vi "PrintScreen.vi"() -> ()   [LabVIEW 2016]
doc: "This code was originally designed to implement a PRINT SCREEN function. If run in its default state, the code simulates a PrintScreen keystroke. When executed, it gives you the option to take a screen capture of the active window (Alt-PrintScreen) or of the entire screen (PrintScreen). I added functionality to choose the keystroke you wish to simulate. It must be noted that the API call for some of the function may or may not cause minor inconvenient responses in the Window's environment. The added options were added solely to show the user how to make various API calls."
uses:
  <vilib>/picture/picture.llb/imagedata.ctl
  user32.dll
panel:
  out "y":u32
  out "x-y":u32
  out "Image":T1(plugin-control)
  in  "Keyboard Stroke 2":T2(ring)=enum."PRINT SCREEN"
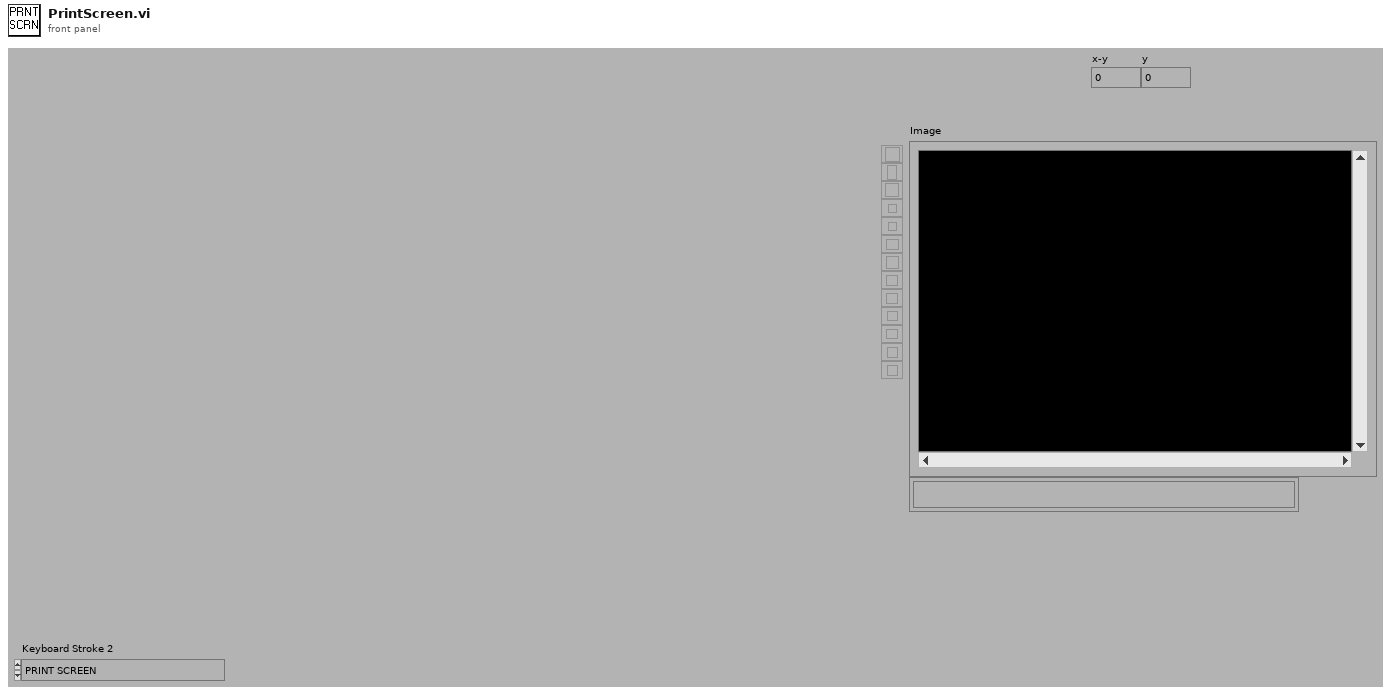
[diagram p1: front panel]
types:
  T1 = typedef "IMAQ Image.ctl" = refnum<image>
  T2 = enum16{"Left Mouse Button", "Right Mouse Button", "Ctrl-Break", "Middle Mouse Button (3-button mice only)", "X1 mouse button (Win2k Only)", "X2 Mouse Button (Win2k Only)", "Undefined (1)", "BACKSPACE", "TAB", "Reserved (1)", "Reserved (2)", "CLEAR", "ENTER", "Undefined (2)", "Undefined (3)", "SHIFT", "CTRL", "ALT", "PAUSE", "CAPS LOCK", "IME Kana mode", "Undefined (4)", "IME Junja mode", "IME final mode", "IME Hanja mode", "IME Kanji mode", "Undefined    ", "ESC", "IME convert", "IME nonconvert", "IME accept", "IME mode change request", "SPACEBAR", "PAGE UP", "PAGE DOWN", "END", "HOME", "LEFT ARROW", "UP ARROW", "RIGHT ARROW", "DOWN ARROW", "SELECT", "PRINT", "EXECUTE", "PRINT SCREEN", "INS", "DEL", "HELP"}
  T3 = typedef "imagedata.ctl" = cluster{"image type":i32, "image depth":i32, "image":u8[], "mask":u8[], "colors":u32[], "Rectangle":cluster{"left":i16, "top":i16, "right":i16, "bottom":i16}}
  T4 = typedef "Image Type" = u32
  T5 = typedef "LVRectTypeDef.ctl" = cluster{"left":i16, "top":i16, "right":i16, "bottom":i16}
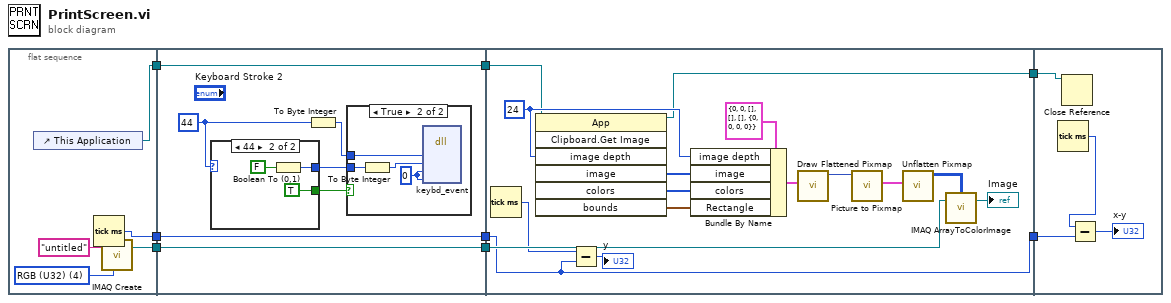
[diagram p0: block diagram]
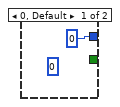
[diagram p3: hidden frame]
diagram:
  n1 = flat-sequence {
    tunnel: [w13] -> w7
    tunnel: [w10] -> w4
    tunnel: [w9] -> w2
    tunnel: [w16] -> w8
    tunnel: w7 -> [w16]
    tunnel: [w15] -> w5
    tunnel: w4 -> [w15]
    tunnel: [w14] -> w3
    tunnel: w2 -> [w14]
    tunnel: w8 -> [w30]
    tunnel: [w30] -> w6
    tunnel: w5 -> [w34]
    tunnel: w3 -> [w33]
    tunnel: [w32] -> w1
    tunnel: w6 -> [w48]
    tunnel: w1 -> [w45]
    frame #0 {
      w12 = T4 4 items=["Grayscale (U8)", "Grayscale (I16)", "Grayscale (SGL)", "Complex (CSG)", "RGB (U32)", "HSL (U32)", "RGB (U64)", "Grayscale (U16)"] ("Image Type")
      n2 = control-ref of="This Application"() -> (w9:refnum<vi>)
      n3 = Tick Count (ms)() -> (millisecond timer value=w13:u32)
      n4 = call "IMAQ Create"("Image Name"="untitled", "Image Type"=w12) -> ("New Image"=w10:T1)  [unwired: 3 in, 1 out]
    }
    frame #1 {
      w17 = 44
      n5 = case shown="44" w17 {
        tunnel: [i16 0 w28] -> w19
        tunnel: [_ TRUE ("T button?")] -> w18
        frame 0, Default {
          (unwired) i16 0
        }
        frame 44 {
          n6 = Boolean To (0,1)(Boolean=FALSE ("T button?")) -> (0, 1=w28:i16)
        }
      }
      n7 = To Byte Integer(number=w17) -> (8bit integer=w20:i8)
      n8 = case shown="True" w18 {
        tunnel: w19 -> [_ w22]
        tunnel: w20 -> [_ w21]
        frame False {
        }
        frame True {
          w23 = 0 ("Input Value")
          n9 = To Byte Integer(number=w22) -> (8bit integer=w24:i8)
          n10 = dll-call lib="user32.dll" fn="keybd_event"(w21, w24, w23, w23) -> ()  [unwired: 7 in, 3 out]
        }
      }
    }
    frame #2 {
      w44 = 24 ("image depth")
      n11 = Tick Count (ms)() -> (millisecond timer value=w31:u32)
      n12 = invoke class="App" method="Clipboard.Get Image"(reference=w33, "image depth"=w44) -> (reference out=w32:refnum<vi>, "image"=w41:u8[], "colors"=w42:u32[], "bounds"=w43:T5)  [unwired: 5 in, 3 out]
      n13 = Subtract(x=w31, y=w30) -> (x-y=→"y":u32)
      n14 = Bundle By Name(cluster=T3 {"image type"=0, "image depth"=0, "image"=[], "mask"=[], "colors"=[], "Rectangle"={"left"=0, "top"=0, "right"=0, "bottom"=0}} ("image data"), "image depth"=w44, "image"=w41, "colors"=w42, "Rectangle"=w43) -> (w39:T3)
      n15 = call <vilib>:"Draw Flattened Pixmap.vi"("image data"=w39) -> ("new picture"=w38:picture)  [unwired: 1 in, 7 out]
      n16 = call <vilib>:"Picture to Pixmap.vi"("picture"=w38) -> ("image data"=w37:T3)  [unwired: 9 in, 1 out]
      n17 = call <vilib>:"Unflatten Pixmap.vi"("image data"=w37) -> ("24-bit pixmap"=w36:u32[][])  [unwired: 4 in, 6 out]
      n18 = call "IMAQ ArrayToColorImage"("Image Pixels (U32)"=w36, "Image"=w34) -> ("Image Out"=→"Image":T1)  [unwired: 3 in, 1 out]
    }
    frame #3 {
      n19 = Tick Count (ms)() -> (millisecond timer value=w47:u32)
      n20 = Close Reference(reference=w45) -> ()  [unwired: 1 in, 1 out]
      n21 = Subtract(x=w47, y=w48) -> (x-y=→"x-y":u32)
    }
  }
